vi "Find Next Location.vi"(1 "Crossed Location":cdb, 2 "Current Location":cdb, 3 "Grid":string[][](array[string])) -> (0 "Next Location":cdb)   [LabVIEW 2020, in "AoC 2023.lvlib"]
uses:
  AoC 2023.lvlib
panel:
  # "|"
  # "-"
  # "L"
  # "J"
  # "7"
  # "F"
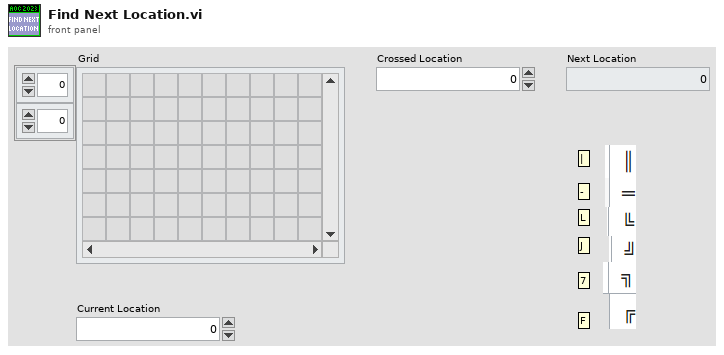
[diagram p1: front panel]
types:
  T1 = cluster{"Up":cdb, "Down":cdb, "Right":cdb, "Left":cdb}
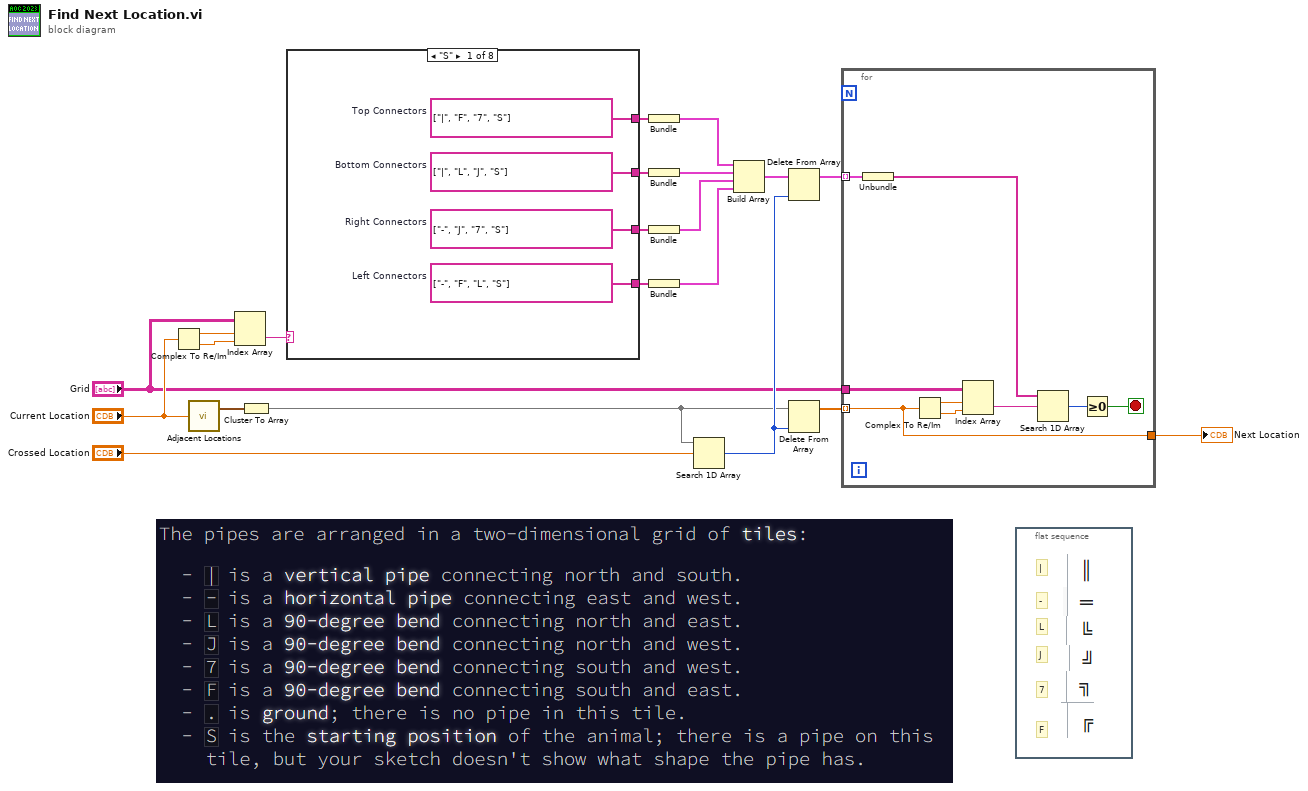
[diagram p0: block diagram]
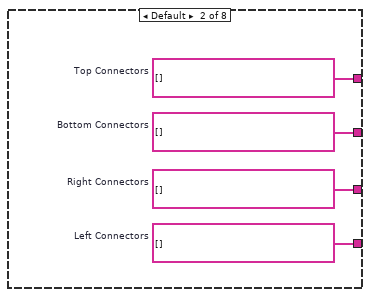
[diagram p2: hidden frame]
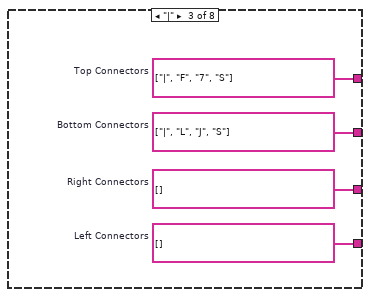
[diagram p3: hidden frame]
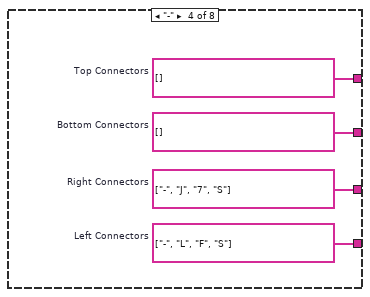
[diagram p4: hidden frame]
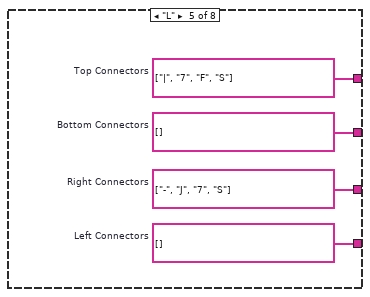
[diagram p5: hidden frame]
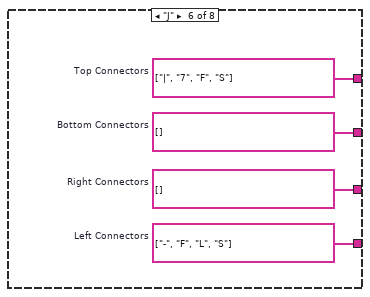
[diagram p6: hidden frame]
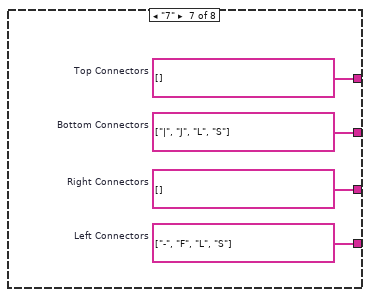
[diagram p7: hidden frame]
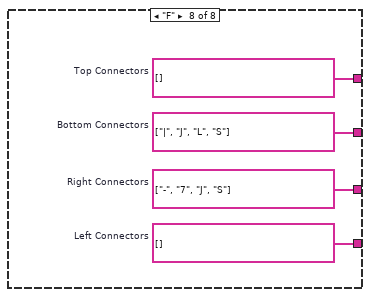
[diagram p8: hidden frame]
diagram:
  n1 = Complex To Re/Im(x + iy="Current Location") -> (x=w4:dbl, y=w5:dbl)
  n2 = call "Adjacent Locations.vi"("Current Location"="Current Location") -> ("4 Adjacent Locations"=w7:T1)  [unwired: 4 in, 1 out]
  n3 = Index Array(array="Grid", index (row)=w4, index (col)=w5) -> (element=w1:string)
  n4 = Cluster To Array(cluster=w7) -> (array=w6:cdb[])
  n5 = case shown="\"S\"" w1 {
    tunnel: [w25 w29 w33 w37 w41 w45 w49 w53] -> w14
    tunnel: [w24 w28 w32 w36 w40 w44 w48 w52] -> w13
    tunnel: [w23 w27 w31 w35 w39 w43 w47 w51] -> w12
    tunnel: [w22 w26 w30 w34 w38 w42 w46 w50] -> w11
    frame "S" {
      w25 = string[] ["-", "F", "L", "S"]  # Left Connectors
      w24 = string[] ["-", "J", "7", "S"]  # Right Connectors
      w23 = string[] ["|", "L", "J", "S"]  # Bottom Connectors
      w22 = string[] ["|", "F", "7", "S"]  # Top Connectors
    }
    frame Default {
      w29 = string[] []  # Left Connectors
      w28 = string[] []  # Right Connectors
      w27 = string[] []  # Bottom Connectors
      w26 = string[] []  # Top Connectors
    }
    frame "|" {
      w33 = string[] []  # Left Connectors
      w32 = string[] []  # Right Connectors
      w31 = string[] ["|", "L", "J", "S"]  # Bottom Connectors
      w30 = string[] ["|", "F", "7", "S"]  # Top Connectors
    }
    frame "-" {
      w37 = string[] ["-", "L", "F", "S"]  # Left Connectors
      w36 = string[] ["-", "J", "7", "S"]  # Right Connectors
      w35 = string[] []  # Bottom Connectors
      w34 = string[] []  # Top Connectors
    }
    frame "L" {
      w41 = string[] []  # Left Connectors
      w40 = string[] ["-", "J", "7", "S"]  # Right Connectors
      w39 = string[] []  # Bottom Connectors
      w38 = string[] ["|", "7", "F", "S"]  # Top Connectors
    }
    frame "J" {
      w45 = string[] ["-", "F", "L", "S"]  # Left Connectors
      w44 = string[] []  # Right Connectors
      w43 = string[] []  # Bottom Connectors
      w42 = string[] ["|", "7", "F", "S"]  # Top Connectors
    }
    frame "7" {
      w49 = string[] ["-", "F", "L", "S"]  # Left Connectors
      w48 = string[] []  # Right Connectors
      w47 = string[] ["|", "J", "L", "S"]  # Bottom Connectors
      w46 = string[] []  # Top Connectors
    }
    frame "F" {
      w53 = string[] []  # Left Connectors
      w52 = string[] ["-", "7", "J", "S"]  # Right Connectors
      w51 = string[] ["|", "J", "L", "S"]  # Bottom Connectors
      w50 = string[] []  # Top Connectors
    }
  }
  n6 = Bundle("Top Connectors"=w11) -> (w15:cluster{"Top Connectors":string[]})  [unwired: 1 in]
  n7 = Bundle("Bottom Connectors"=w12) -> (w16:cluster{"Bottom Connectors":string[]})  [unwired: 1 in]
  n8 = Bundle("Right Connectors"=w13) -> (w17:cluster{"Right Connectors":string[]})  [unwired: 1 in]
  n9 = Bundle("Left Connectors"=w14) -> (w18:cluster{"Left Connectors":string[]})  [unwired: 1 in]
  n10 = Search 1D Array(1D array=w6, element="Crossed Location") -> (index of element=w8:i32)  [unwired: 1 in]
  n11 = Build Array(w15, w16, w17, w18) -> (w10:cluster{"Left Connectors":string[]}[])
  n12 = Delete From Array(array=w10, index=w8) -> (array with subset deleted=w9:cluster{"Left Connectors":string[]}[])  [unwired: 1 in, 1 out]
  n13 = Delete From Array(array=w6, index=w8) -> (array with subset deleted=w20:cdb[])  [unwired: 1 in, 1 out]
  n14 = for {
    tunnel: "Grid" -> [w62]
    tunnel: w9 -> [w57] mode=indexing
    tunnel: [w54] -> w19
    tunnel: w20 -> [w54] mode=indexing
    stop <- w55 stop-if-true
    n15 = Unbundle(w57) -> ("Left Connectors"=w56:string[])
    n16 = Complex To Re/Im(x + iy=w54) -> (x=w61:dbl, y=w60:dbl)
    n17 = Index Array(array=w62, index (row)=w61, index (col)=w60) -> (element=w59:string)
    n18 = Search 1D Array(1D array=w56, element=w59) -> (index of element=w58:i32)  [unwired: 1 in]
    n19 = Greater Or Equal To 0?(x=w58) -> (x >= 0?=w55:bool)
  }
  "Next Location" <- w19
  n20 = flat-sequence {
    frame #0 {
      # "F"
      # "7"
      # "J"
      # "L"
      # "-"
      # "|"
    }
  }
